vi "RegisterPublisherByType.vi"(6 "Lock Topic":bool, 7 "Event":refnum<class "Message Interface.lvclass">, 8 "error in (no error)":errorcluster, 11 "EDA Message Broker Interface Ref in":refnum<class "EDA Message Broker Interface Ref.lvclass">=refnum) -> (0 "error out":errorcluster, 3 "EDA Message Broker Interface Ref out":refnum<class "EDA Message Broker Interface Ref.lvclass">, 4 "Locked?":bool, 5 "Transport":refnum<class "Message Transport Queue.lvclass">)   [LabVIEW 2016, in "Stream Mediator.lvlib" / "EDA Message Broker Interface Ref.lvclass"]
doc: "--\nCopyright © 2017 Composed SystemsI All rights reserved.\n\nAuthor: Jon McBee <jon.mcbee@composed.io>\n\nThis library is provided \"AS IS\" ,WITHOUT WARRANTIES OR\nCONDITIONS OF ANY KIND, either express or implied.\n\nComposed Systems -- composed.io\n\nStream 0.0.1.1\nJon McBee - Composed Systems\nCopyright (c) 2017, Composed Systems"
uses:
  <userlib>/Composed Systems/Stream/Mediator/Classes/EDA Message Broker Interface Ref/EDA Message Broker Interface Ref.lvclass
  C:/Program Files (x86)/National Instruments/LabVIEW 2016/user.lib/Composed Systems/Stream/Mediator/Classes/Message Broker Interface Ref/Message Broker Interface Ref.lvclass
  <userlib>/Composed Systems/Stream/Mediator/Classes/Message Transport Queue/Message Transport Queue.lvclass
  <userlib>/Composed Systems/Stream/Mediator/Classes/Message Interface/Message Interface.lvclass
  <userlib>/Composed Systems/Stream/Mediator/Classes/Message Broker/Message Broker.lvclass
  <userlib>/Composed Systems/Stream/Mediator/Classes/Message Broker Interface Ref/Message Broker Interface Ref.lvclass
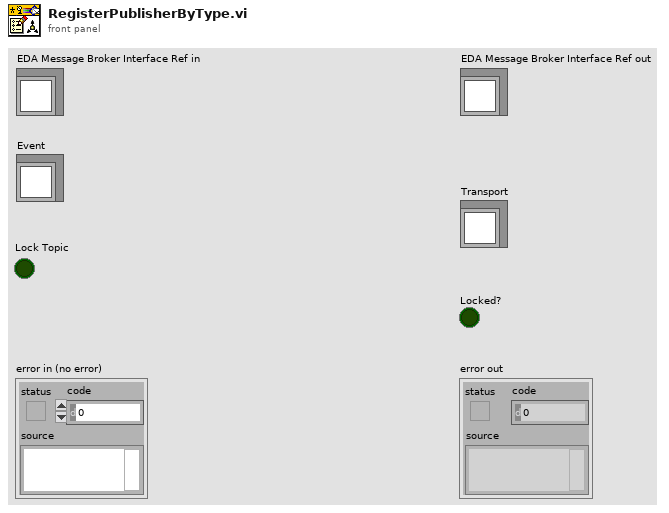
[diagram p1: front panel]
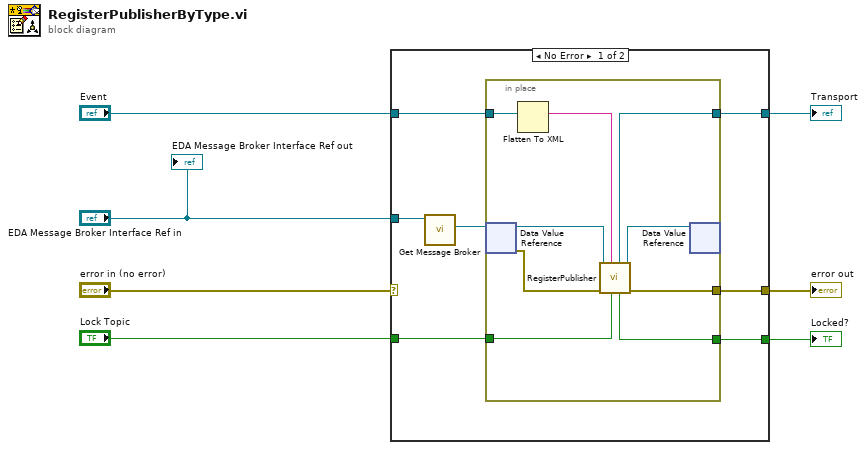
[diagram p0: block diagram]
diagram:
  n1 = case shown="No Error" "error in (no error)" {
    selector: "error in (no error)" -> [_ w24]
    tunnel: "EDA Message Broker Interface Ref in" -> [w14 _]
    tunnel: "Event" -> [w12 _]
    tunnel: [w11 _] -> w4
    tunnel: [w10 w24] -> w3
    tunnel: "Lock Topic" -> [w9 _]
    tunnel: [w8 _] -> w1
    frame No Error {
      n2 = call <userlib>:"Get Message Broker.vi"("Message Broker Interface Ref in"=w14) -> ("Broker"=w13:refnum<data-value>)  [unwired: 8 in, 2 out]
      n3 = in-place {
        in-place-border: w12 -> [w22]
        in-place-border: [w20] -> w11
        in-place-border: [w18] -> w10
        in-place-border: w9 -> [w16]
        in-place-border: [w15] -> w8
        n4 = in-place-dvr #1(w13) -> (w23:refnum<class "Message Broker.lvclass">, w17:errorcluster)
        n5 = Flatten To XML(anything=w22) -> (xml string=w21:string)
        n6 = call <userlib>:"RegisterPublisher.vi"("1:M"=w16, "Topic Name"=w21, "error in (no error)"=w17, "Message Broker in"=w23) -> ("error out"=w18:errorcluster, "Message Broker out"=w19:refnum<class "Message Broker.lvclass">, "Locked?"=w15:bool, "Transport"=w20:refnum<class "Message Transport Queue.lvclass">)  [unwired: 3 in, 1 out]
        n7 = in-place-dvr #1(w19) -> ()  [unwired: 2 out]
      }
    }
    frame Error {
    }
  }
  "error out" <- w3
  "Transport" <- w4
  "Locked?" <- w1
  "EDA Message Broker Interface Ref out" <- "EDA Message Broker Interface Ref in"
